vi "filter_temp_pot.vi"(11 "Datos Leídos T y P 2":string[](array[string])) -> (2 "Curva de potencia":cluster{"Ramp Pattern":dbl[], u32[]}(graph), 3 "Curva de temperatura":cluster{"Ramp Pattern":dbl[], u32[]}(graph))   [LabVIEW 2021]
uses:
  <vilib>/Analysis/1siggen.llb/Ramp Pattern by Delta.vi
  <vilib>/Analysis/NI_AALBase.lvlib
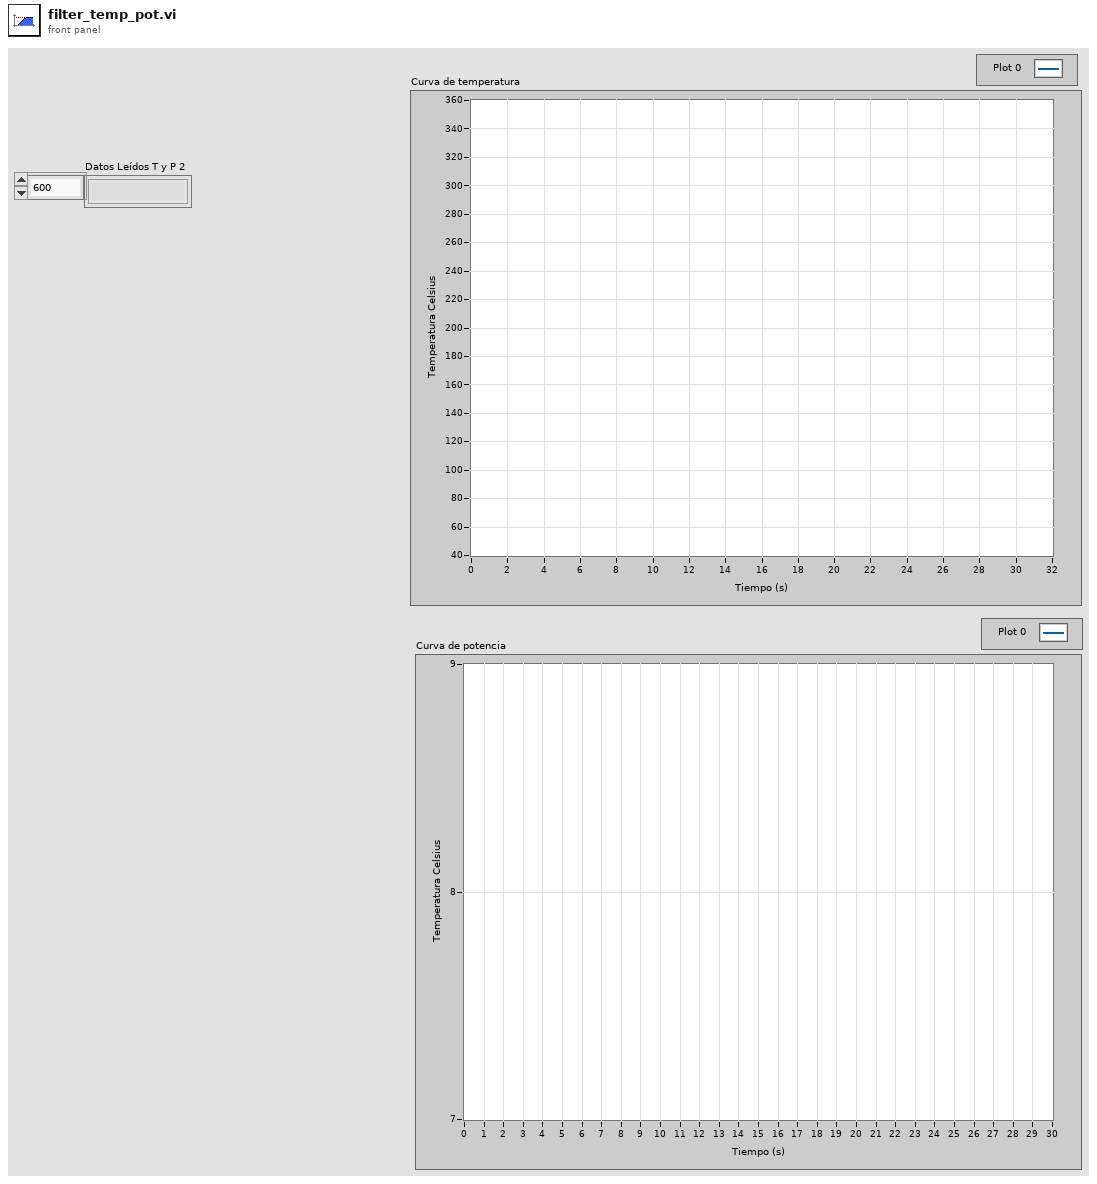
[diagram p1: front panel]
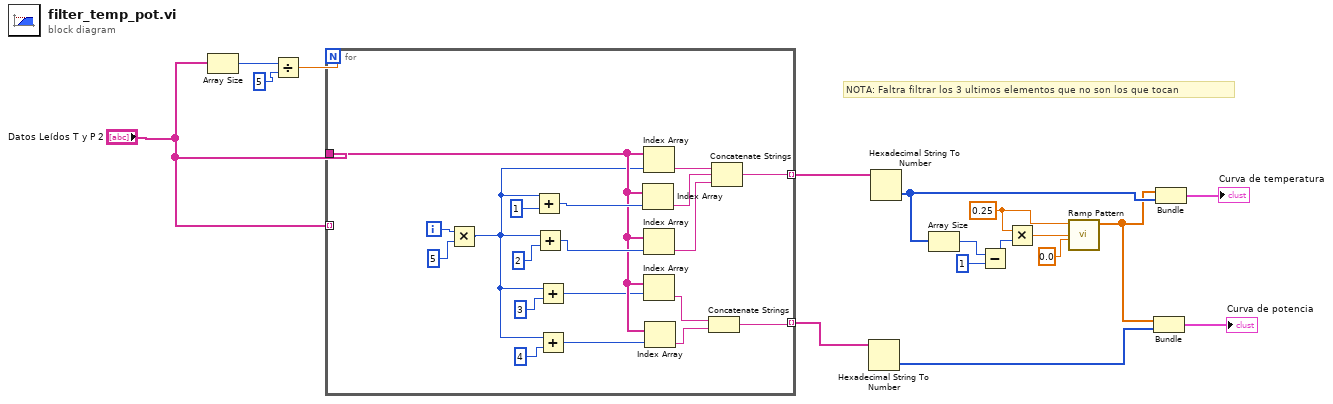
[diagram p0: block diagram]
diagram:
  w10 = 0.25 ("delta")
  # "NOTA: Faltra filtrar los 3 ultimos elementos que no son los que tocan"
  n1 = Array Size(array="Datos Leídos T y P 2") -> (size(s)=w12:i32)
  n2 = Divide(x=w12, y=5) -> (x/y=w14:dbl)
  n3 = for {
    N: w14 -> [_]
    tunnel: "Datos Leídos T y P 2" -> [_] mode=indexing
    tunnel: "Datos Leídos T y P 2" -> [w26]
    tunnel: [w33] -> w15 mode=indexing
    tunnel: [w18] -> w5 mode=indexing
    i -> [w28]
    n4 = Multiply(x=w28, y=5) -> (x*y=w25:i32)
    n5 = Add(x=w25, y=1) -> (x+y=w30:i32)
    n6 = Add(x=w25, y=2) -> (x+y=w29:i32)
    n7 = Add(x=w25, y=3) -> (x+y=w22:i32)
    n8 = Add(x=w25, y=4) -> (x+y=w21:i32)
    n9 = Index Array(array=w26, index=w30) -> (element=w35:string)
    n10 = Index Array(array=w26, index=w25) -> (element=w36:string)
    n11 = Index Array(array=w26, index=w29) -> (element=w34:string)
    n12 = Index Array(array=w26, index=w22) -> (element=w20:string)
    n13 = Index Array(array=w26, index=w21) -> (element=w19:string)
    n14 = Concatenate Strings(w20, w19) -> (w18:string)
    n15 = Concatenate Strings(w36, w35, w34) -> (w33:string)
  }
  n16 = Hexadecimal String To Number(string=w5) -> (number=w3:u32[])  [unwired: 2 in, 1 out]
  n17 = Hexadecimal String To Number(string=w15) -> (number=w11:u32[])  [unwired: 2 in, 1 out]
  n18 = Array Size(array=w11) -> (size(s)=w8:i32)
  n19 = Subtract(x=w8, y=1) -> (x-y=w6:i32)
  n20 = Multiply(x=w10, y=w6) -> (x*y=w9:dbl)
  n21 = call-poly <vilib>:"Ramp Pattern.vi"("start"=0.0, "end"=w9, "delta"=w10) -> ("Ramp Pattern"=w4:dbl[])  [unwired: 6 in, 2 out]
  n22 = Bundle("Ramp Pattern"=w4, w3) -> (→"Curva de potencia":cluster{"Ramp Pattern":dbl[], u32[]})  [unwired: 1 in]
  n23 = Bundle("Ramp Pattern"=w4, w11) -> (→"Curva de temperatura":cluster{"Ramp Pattern":dbl[], u32[]})  [unwired: 1 in]
